vi "solar_voy_def HS_DATA.vi"(8 "Error Source":string, 9 "PACKET_DATA":string, 10 "PACKET":string, 11 "TARGET":string) -> (3 "HS_DATA":string)   [LabVIEW 2018]
doc: "This packs the HANDSHAKE DATA item field. \n\nHANDSHAKE DATA item:\nU8: <target_name_length>\nSTR: <target_name>\nU8: <packet_name_length>\nSTR: <packet_name>\nI32: <packet_data_size>\nSTR: <packet_data>\nI32: <error_source_size>\nSTR: <error_source>"
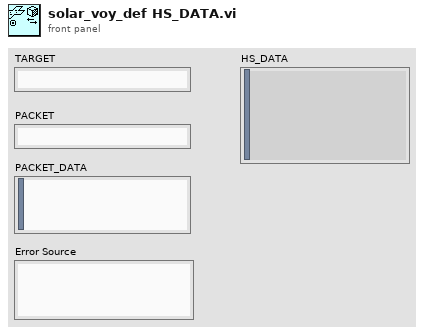
[diagram p1: front panel]
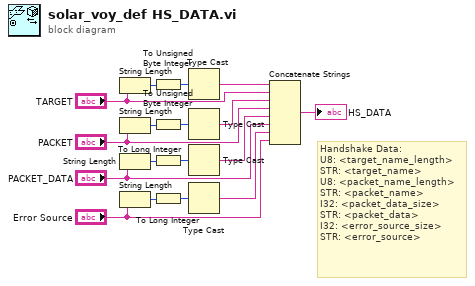
[diagram p0: block diagram]
diagram:
  # "Handshake Data:\nU8: <target_name_length>\nSTR: <target_name>\nU8: <packet_name_length>\nSTR: <packet_name>\nI32: <packet_data_size>\nSTR: <packet_data>\nI32: <error_source_size>\nSTR: <error_source>"
  n1 = String Length(string="TARGET") -> (length=w10:i32)
  n2 = String Length(string="PACKET") -> (length=w6:i32)
  n3 = String Length(string="PACKET_DATA") -> (length=w4:i32)
  n4 = String Length(string="Error Source") -> (length=w2:i32)
  n5 = To Unsigned Byte Integer(number=w10) -> (unsigned 8bit integer=w9:u8)
  n6 = To Unsigned Byte Integer(number=w6) -> (unsigned 8bit integer=w7:u8)
  n7 = To Long Integer(number=w4) -> (32bit integer=w11:i32)
  n8 = To Long Integer(number=w2) -> (32bit integer=w12:i32)
  n9 = Type Cast(x=w9) -> (*(type *) &x=w8:string)  [unwired: 1 in]
  n10 = Type Cast(x=w7) -> (*(type *) &x=w5:string)  [unwired: 1 in]
  n11 = Type Cast(x=w11) -> (*(type *) &x=w3:string)  [unwired: 1 in]
  n12 = Type Cast(x=w12) -> (*(type *) &x=w1:string)  [unwired: 1 in]
  n13 = Concatenate Strings(w8, "TARGET", w5, "PACKET", w3, "PACKET_DATA", w1, "Error Source") -> (→"HS_DATA":string)
